vi "Control_Moved.vi"(8 "error in (no error)":errorcluster, 11 "Camera_Scan_Controller.lvclass":refnum<class "Camera_Scan_Controller.lvclass">) -> (0 "error out":errorcluster, 3 "Camera_Scan_Controller.lvlib:Camera_Scan_Controller.lvclass":refnum<class "Camera_Scan_Controller.lvclass">)   [LabVIEW 2023, in "Camera_Scan_Controller.lvlib" / "Camera_Scan_Controller.lvclass"]
uses:
  Camera_Scan_Controller.lvclass
  Camera_Scan_Controller.lvclass/Camera_Scan_Controller.ctl
  <vilib>/ActorFramework/Message Enqueuer/Message Enqueuer.lvclass/Message Enqueuer.ctl
  <vilib>/ActorFramework/Message Enqueuer/Enqueue.vi
  Camera_Scan_Controller Messages/Acquisition Done Msg/Acquisition Done Msg.lvclass
  C:/Program Files/National Instruments/LabVIEW 2023/vi.lib/ActorFramework/Message/Message.lvclass
  UIs/Camera_Controller/Camera_Controller/TopControllerComm Messages/External_Move Msg/External_Move Msg.lvclass
  <vilib>/ActorFramework/Message Priority Queue/Priority Enqueue.vi
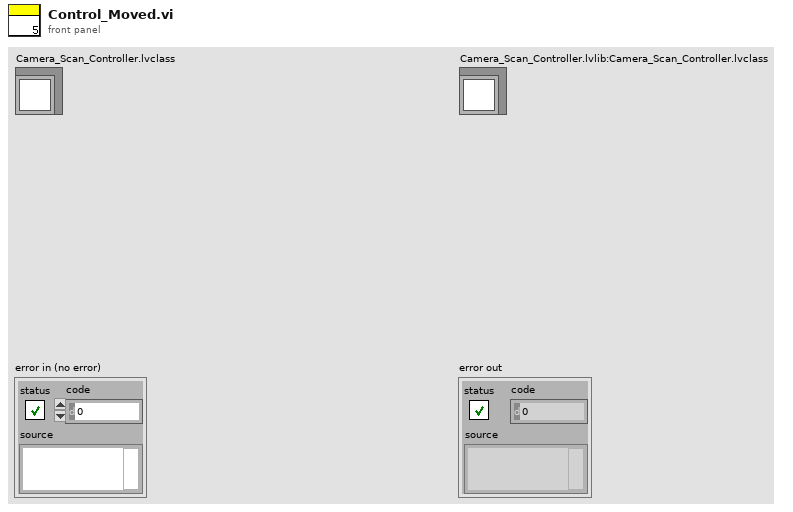
[diagram p1: front panel]
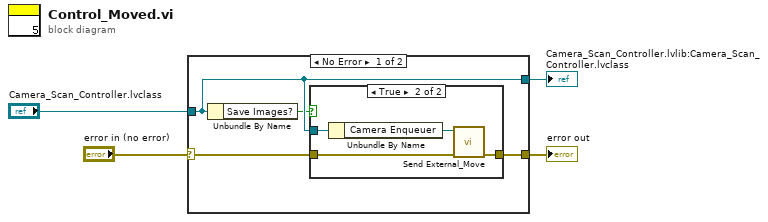
[diagram p0: block diagram]
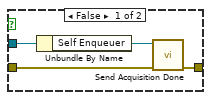
[diagram p2: hidden frame]
diagram:
  n1 = case shown="No Error" "error in (no error)" {
    selector: "error in (no error)" -> [w8 w18]
    tunnel: [w7 w18] -> w3
    tunnel: [w6 w17] -> w1
    tunnel: "Camera_Scan_Controller.lvclass" -> [w6 w17]
    frame No Error {
      n2 = Unbundle By Name(w6) -> ("Save Images?"=w5:bool)
      n3 = case shown="True" w5 {
        tunnel: w6 -> [w12 w16]
        tunnel: w8 -> [w10 w13]
        tunnel: [w9 w14] -> w7
        frame False {
          n4 = Unbundle By Name(w12) -> ("Self Enqueuer"=w11:refnum<class "Message Enqueuer.lvclass">)
          n5 = call "Send Acquisition Done.vi"("error in (no error)"=w10, "Message Enqueuer"=w11) -> ("error out"=w9:errorcluster)  [unwired: 8 in, 1 out]
        }
        frame True {
          n6 = Unbundle By Name(w16) -> ("Camera Enqueuer"=w15:refnum<class "Message Enqueuer.lvclass">)
          n7 = call "Send External_Move.vi"("error in (no error)"=w13, "Message Enqueuer"=w15) -> ("error out"=w14:errorcluster)  [unwired: 8 in, 1 out]
        }
      }
    }
    frame Error {
    }
  }
  "error out" <- w3
  "Camera_Scan_Controller.lvlib:Camera_Scan_Controller.lvclass" <- w1
